vi "pickVSSTeam.vi"(0 "Ally in":refnum<class "Ally.lvclass">, 1 "OldVSSTeam":refnum<class "Ally.lvclass">, 2 "RobotRef":refnum<class "Robot.lvclass">[](array[class]), 3 "error in (no error)":errorcluster, 4 "Game":refnum<class "Game.lvclass">) -> (7 "Ally out":refnum<class "Ally.lvclass">, 8 "RobotRef Out":refnum<class "Robot.lvclass">[](array[class]), 10 "error out":errorcluster)   [LabVIEW 2020, in "Ally.lvclass"]
uses:
  Ally.lvclass
  C:/Users/lucio/Desktop/Horie/ROBOIME/VSS_AI/Team_class/Team.lvclass
  Game_class/Game.lvclass
  Robot_class/Robot.lvclass
  Utilities_class/Utilities.lvclass
  Game_class/Game.lvclass/Game.ctl
  Team_class/Team.lvclass/Team.ctl
  Game_class/Read Parameters.lvclass.vi
  Game_class/Read BallRef.vi
  Team_class/Write RobotRef.vi
  Parameters_class/Parameters.lvclass
  Ball_class/Ball.lvclass
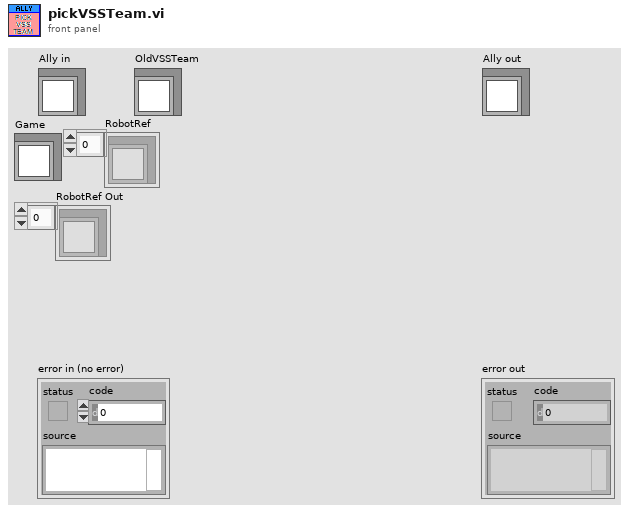
[diagram p1: front panel]
types:
  T1 = cluster{"Robots ids":cluster{"Goalie":enum16{"auto", "5", "4", "3", "2", "1", "0"}, "Attacker":enum16{"auto", "5", "4", "3", "2", "1", "0"}, "Defender":enum16{"auto", "5", "4", "3", "2", "1", "0"}}}
  T2 = cluster{"Goalie":enum16{"auto", "5", "4", "3", "2", "1", "0"}, "Attacker":enum16{"auto", "5", "4", "3", "2", "1", "0"}, "Defender":enum16{"auto", "5", "4", "3", "2", "1", "0"}}
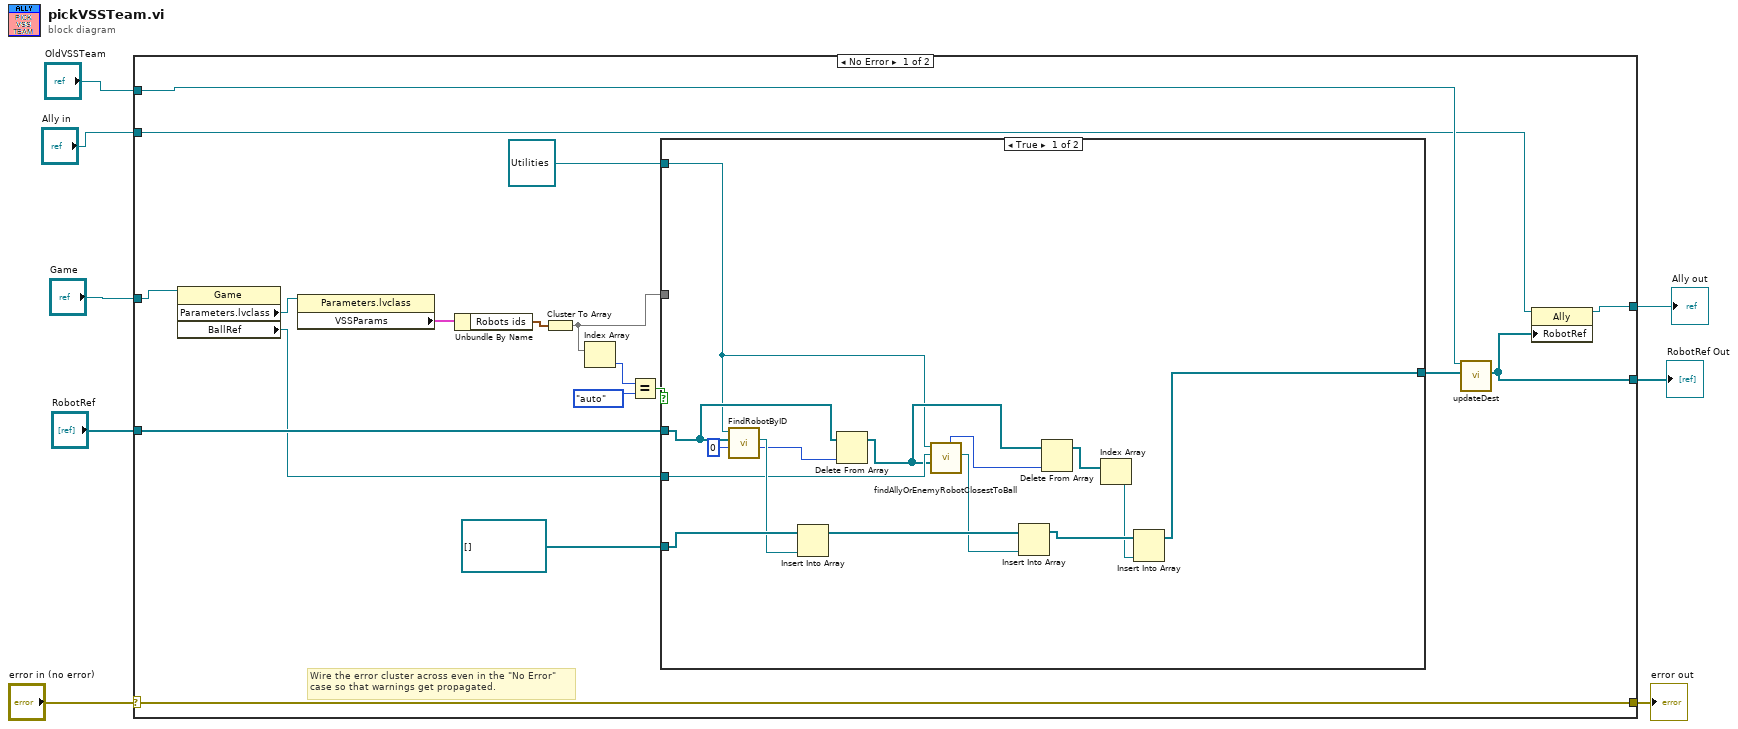
[diagram p0: block diagram]
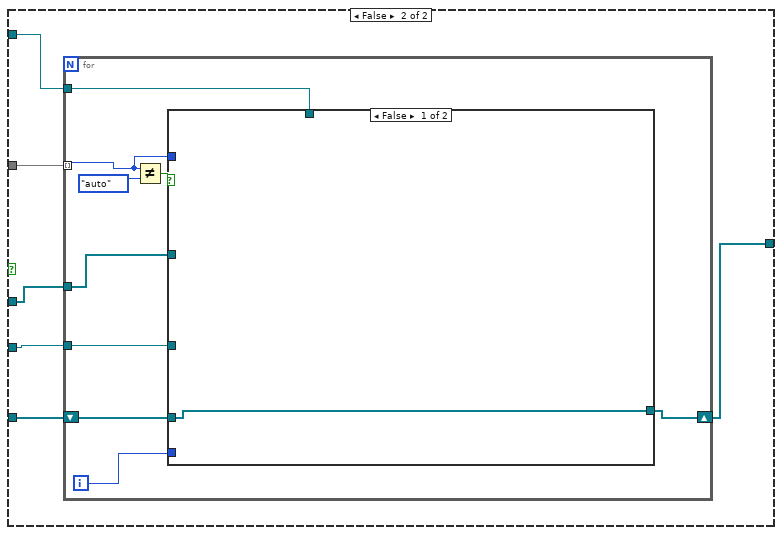
[diagram p2: hidden frame]
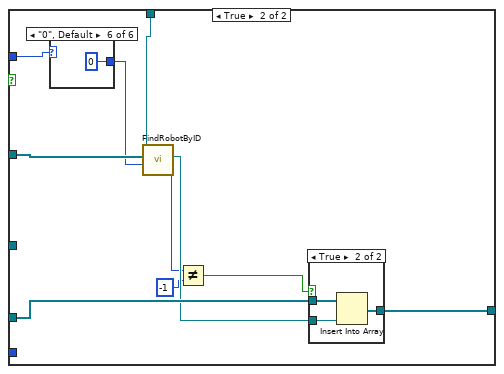
[diagram p3: hidden frame]
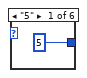
[diagram p4: hidden frame]
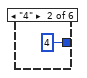
[diagram p5: hidden frame]
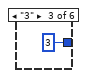
[diagram p6: hidden frame]
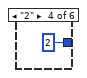
[diagram p7: hidden frame]
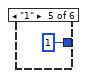
[diagram p8: hidden frame]
diagram:
  n1 = case shown="No Error" "error in (no error)" {
    selector: "error in (no error)" -> [w26 w78]
    tunnel: [w26 w78] -> w7
    tunnel: "Game" -> [w25 _]
    tunnel: "OldVSSTeam" -> [w22 _]
    tunnel: "Ally in" -> [w21 _]
    tunnel: [w20 _] -> w3
    tunnel: [w19 _] -> w2
    tunnel: "RobotRef" -> [w18 _]
    frame No Error {
      # "Wire the error cluster across even in the \"No Error\"\ncase so that warnings get propagated."
      n2 = property class="Game"(reference=w25) -> ("Parameters.lvclass"=w24:refnum<class "Parameters.lvclass">, "BallRef"=w14:refnum<class "Ball.lvclass">)  [unwired: 1 in, 2 out]
      n3 = property class="Parameters.lvclass"(reference=w24) -> ("VSSParams"=w23:T1)  [unwired: 1 in, 2 out]
      n4 = Unbundle By Name(w23) -> ("Robots ids"=w13:T2)
      n5 = Cluster To Array(cluster=w13) -> (array=w12:enum16{"auto", "5", "4", "3", "2", "1", "0"}[])
      n6 = Index Array(array=w12) -> (element=w10:enum16{"auto", "5", "4", "3", "2", "1", "0"})  [unwired: 1 in]
      n7 = Equal?(x=w10, y=enum16{"auto", "5", "4", "3", "2", "1", "0"}."auto") -> (x = y?=w9:bool)
      n8 = case shown="True" w9 {
        tunnel: w18 -> [w38 w47]
        tunnel: refnum<class "Utilities.lvclass"> refnum ("Utilities in") -> [w27 w46]
        tunnel: refnum<class "Robot.lvclass">[] [] ("RobotRef") -> [w40 w45]
        tunnel: [w28 w44] -> w15
        tunnel: w14 -> [w36 w43]
        tunnel: w12 -> [_ w42]
        frame True {
          n9 = call-dynamic "FindRobotByID.vi"("id"=0, "RobotRef"=w38, "Utilities in"=w27) -> ("index"=w37:i32, "Robot"=w39:refnum<class "Robot.lvclass">)  [unwired: 5 in, 2 out]
          n10 = Insert Into Array(array=w40, new element=w39) -> (w35:refnum<class "Robot.lvclass">[])  [unwired: 1 in]
          n11 = Delete From Array(array=w38, index=w37) -> (array with subset deleted=w33:refnum<class "Robot.lvclass">[])  [unwired: 1 in, 1 out]
          n12 = call "findAllyOrEnemyRobotClosestToBall.vi"("Ally/Enemy Robots"=w33, "Ball"=w36, "Utilities in"=w27) -> ("Robot"=w34:refnum<class "Robot.lvclass">, "Numeric"=w32:i32)  [unwired: 4 in, 3 out]
          n13 = Insert Into Array(array=w35, new element=w34) -> (w30:refnum<class "Robot.lvclass">[])  [unwired: 1 in]
          n14 = Delete From Array(array=w33, index=w32) -> (array with subset deleted=w31:refnum<class "Robot.lvclass">[])  [unwired: 1 in, 1 out]
          n15 = Index Array(array=w31) -> (element=w29:refnum<class "Robot.lvclass">)  [unwired: 1 in]
          n16 = Insert Into Array(array=w30, new element=w29) -> (w28:refnum<class "Robot.lvclass">[])  [unwired: 1 in]
        }
        frame False {
          n17 = for {
            tunnel: w42 -> [w50] mode=indexing
            tunnel: w46 -> [w55]
            shift-right: [w49] -> w44
            shift-left: w45 -> [w51]
            tunnel: w43 -> [w48]
            tunnel: w47 -> [w56]
            i -> [w52]
            n18 = Not Equal?(x=w50, y=enum16{"auto", "5", "4", "3", "2", "1", "0"}."auto") -> (x != y?=w53:bool)
            n19 = case shown="False" w53 {
              tunnel: w56 -> [_ w66]
              tunnel: w55 -> [_ w67]
              tunnel: [w57 w63] -> w49
              tunnel: w52 -> [_ _]
              tunnel: w51 -> [w57 w65]
              tunnel: w50 -> [_ w59]
              tunnel: w48 -> [_ _]
              frame False {
              }
              frame True {
                n20 = case shown="\"0\", Default" w59 {
                  tunnel: [5 4 3 2 1 0] -> w58
                  frame "5" {
                  }
                  frame "4" {
                  }
                  frame "3" {
                  }
                  frame "2" {
                  }
                  frame "1" {
                  }
                  frame "0", Default {
                  }
                }
                n21 = call-dynamic "FindRobotByID.vi"("id"=w58, "RobotRef"=w66, "Utilities in"=w67) -> ("index"=w61:i32, "Robot"=w64:refnum<class "Robot.lvclass">)  [unwired: 5 in, 2 out]
                n22 = Not Equal?(x=w61, y=-1 ("index")) -> (x != y?=w60:bool)
                n23 = case shown="True" w60 {
                  tunnel: w65 -> [w74 w77]
                  tunnel: w64 -> [_ w76]
                  tunnel: [w74 w75] -> w63
                  frame False {
                  }
                  frame True {
                    n24 = Insert Into Array(array=w77, new element=w76) -> (w75:refnum<class "Robot.lvclass">[])  [unwired: 1 in]
                  }
                }
              }
            }
          }
        }
      }
      n25 = call "updateDest.vi"("NewAllyRobots"=w15, "LastAlly"=w22) -> ("NewAllyRobotsUpdated"=w19:refnum<class "Robot.lvclass">[])  [unwired: 7 in, 2 out]
      n26 = property class="Ally"(reference=w21, "RobotRef"=w19) -> (reference out=w20:refnum<class "Ally.lvclass">)  [unwired: 1 in, 1 out]
    }
    frame Error {
    }
  }
  "error out" <- w7
  "Ally out" <- w3
  "RobotRef Out" <- w2
